vi "Secondary Xbox.vi"(10 "Secondary":T3, 11 "Dash Data In":T2={"Joy Stick"={"Primary"={"Buttons"={"A"=FALSE, "B"=FALSE, "X"=FALSE, "Y"=FALSE, "Left Bumper"=FALSE, "Right Bumper"=FALSE, "Back"=FALSE, "Start"=FALSE, "Left Thumbstick"=FALSE, "Right Thumbstick"=FALSE}, "Axes"={"Left Stick X "=0.0, "Left Stick Y"=0.0, "Triggers"=-0.0, "Right Stick X"=0.0, "Right Stick Y"=0.0, "D-Pad X"=0.0}}, "Secondary"={"Buttons"={"A"=FALSE, "B"=FALSE, "X"=FALSE, "Y"=FALSE, "Left Bumper"=FALSE, "Right Bumper"=FALSE, "Back"=FALSE, "Start"=FALSE, "Left Thumbstick"=FALSE, "Right Thumbstick"=FALSE}, "Axes"={"Left Stick X "=0.0, "Left Stick Y"=0.0, "Triggers"=0.0, "Right Stick X"=0.0, "Right Stick Y"=0.0, "D-Pad X"=0.0}}}, "Shooter"={"RPM Current"=0.0, "RPM Set"=0.0, "In Range?"=FALSE}, "Arm"={"Arm Current"=0.0, "Arm Set"=0.0, "At Position?"=FALSE, "Reset Encoder"=FALSE}, "Drive"={"Right"=0.0, "Left"=0.0}, "Climb State"=enum."Arm Attach", "Change Retical"=FALSE, "Solenoids"={"Robot Angle"=enum."Off", "Shooter Angle"=enum."Off", "Arm Lock"=enum."Off"}, "Shooter Speeds"=[]}) -> (3 "Dash Data Out 2":T2={"Joy Stick"={"Primary"={"Buttons"={"A"=FALSE, "B"=FALSE, "X"=FALSE, "Y"=FALSE, "Left Bumper"=FALSE, "Right Bumper"=FALSE, "Back"=FALSE, "Start"=FALSE, "Left Thumbstick"=FALSE, "Right Thumbstick"=FALSE}, "Axes"={"Left Stick X "=0.0, "Left Stick Y"=0.0, "Triggers"=-0.0, "Right Stick X"=0.0, "Right Stick Y"=0.0, "D-Pad X"=0.0}}, "Secondary"={"Buttons"={"A"=FALSE, "B"=FALSE, "X"=FALSE, "Y"=FALSE, "Left Bumper"=FALSE, "Right Bumper"=FALSE, "Back"=FALSE, "Start"=FALSE, "Left Thumbstick"=FALSE, "Right Thumbstick"=FALSE}, "Axes"={"Left Stick X "=0.0, "Left Stick Y"=0.0, "Triggers"=0.0, "Right Stick X"=0.0, "Right Stick Y"=0.0, "D-Pad X"=0.0}}}, "Shooter"={"RPM Current"=0.0, "RPM Set"=0.0, "In Range?"=FALSE}, "Arm"={"Arm Current"=0.0, "Arm Set"=0.0, "At Position?"=FALSE, "Reset Encoder"=FALSE}, "Drive"={"Right"=0.0, "Left"=0.0}, "Climb State"=enum."Arm Attach", "Change Retical"=FALSE, "Solenoids"={"Robot Angle"=enum."Off", "Shooter Angle"=enum."Off", "Arm Lock"=enum."Off"}, "Shooter Speeds"=[]})   [LabVIEW 2012]
uses:
  <vilib>/Rock Robotics/WPI/Solenoid/WPI_SolenoidValue.ctl
types:
  T1 = typedef "WPI_SolenoidValue.ctl" = enum16{"Off", "On", "Forward", "Reverse"}
  T2 = cluster{"Joy Stick":cluster{"Primary":cluster{"Buttons":cluster{"A":bool, "B":bool, "X":bool, "Y":bool, "Left Bumper":bool, "Right Bumper":bool, "Back":bool, "Start":bool, "Left Thumbstick":bool, "Right Thumbstick":bool}, "Axes":cluster{"Left Stick X ":dbl, "Left Stick Y":dbl, "Triggers":dbl, "Right Stick X":dbl, "Right Stick Y":dbl, "D-Pad X":dbl}}, "Secondary":cluster{"Buttons":cluster{"A":bool, "B":bool, "X":bool, "Y":bool, "Left Bumper":bool, "Right Bumper":bool, "Back":bool, "Start":bool, "Left Thumbstick":bool, "Right Thumbstick":bool}, "Axes":cluster{"Left Stick X ":dbl, "Left Stick Y":dbl, "Triggers":dbl, "Right Stick X":dbl, "Right Stick Y":dbl, "D-Pad X":dbl}}}, "Shooter":cluster{"RPM Current":dbl, "RPM Set":dbl, "In Range?":bool}, "Arm":cluster{"Arm Current":dbl, "Arm Set":dbl, "At Position?":bool, "Reset Encoder":bool}, "Drive":cluster{"Right":dbl, "Left":dbl}, "Climb State":enum16{"Arm Wait", "Arm Up", "Arm Down", "Arm Attach"}, "Change Retical":bool, "Solenoids":cluster{"Robot Angle":T1, "Shooter Angle":T1, "Arm Lock":T1}, "Shooter Speeds":dbl[]}
  T3 = cluster{"Buttons":cluster{"A":bool, "B":bool, "X":bool, "Y":bool, "Left Bumper":bool, "Right Bumper":bool, "Back":bool, "Start":bool, "Left Thumbstick":bool, "Right Thumbstick":bool}, "Axes":cluster{"Left Stick X ":dbl, "Left Stick Y":dbl, "Triggers":dbl, "Right Stick X":dbl, "Right Stick Y":dbl, "D-Pad X":dbl}}
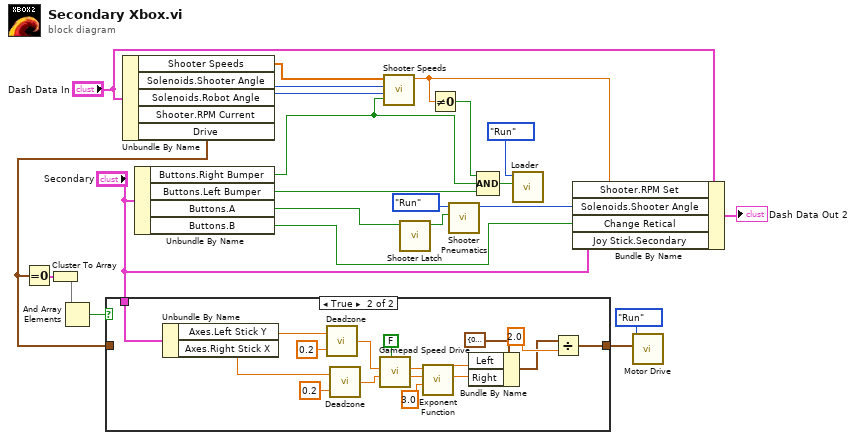
[diagram p0: block diagram]
diagram:
  n1 = Unbundle By Name("Dash Data In") -> ("Shooter Speeds"=w17:dbl[], "Solenoids.Shooter Angle"=w14:T1, "Solenoids.Robot Angle"=w16:T1, "Drive"=w8:cluster{"Right":dbl, "Left":dbl})  [unwired: 1 out]
  n2 = Equal To 0?(x=w8) -> (x = 0?=w9:cluster{"Right":bool, "Left":bool})
  n3 = Cluster To Array(cluster=w9) -> (array=w7:bool[])
  n4 = And Array Elements(Boolean array=w7) -> (logical AND=w6:bool)
  n5 = case shown="True" w6 {
    tunnel: "Secondary" -> [_ w30]
    tunnel: [w24 w26] -> w10
    tunnel: w8 -> [w24 _]
    frame False {
    }
    frame True {
      n6 = Unbundle By Name(w30) -> ("Axes.Left Stick Y"=w29:dbl, "Axes.Right Stick X"=w28:dbl)
      n7 = call "Deadzone.vi"("Deadzone"=0.2, "Input"=w29) -> ("Output"=w37:dbl)
      n8 = call "Deadzone.vi"("Deadzone"=0.2, "Input"=w28) -> ("Output"=w35:dbl)
      n9 = call "Gamepad Speed Drive.vi"("Quick Turn"=FALSE, "Turn"=w35, "Speed"=w37) -> ("Right Output"=w40:dbl, "Left Output"=w41:dbl)  [unwired: 7 in]
      n10 = call "Exponent Function.vi"("Exponent"=3.0, "Left In"=w40, "Right In"=w41) -> ("Right Out"=w32:dbl, "Left Out"=w33:dbl)  [unwired: 7 in]
      n11 = Bundle By Name(cluster=cluster{"Right":dbl, "Left":dbl} {"Right"=0.0, "Left"=0.0} ("Motor"), "Left"=w33, "Right"=w32) -> (w27:cluster{"Right":dbl, "Left":dbl})
      n12 = Divide(x=w27, y=2.0) -> (x/y=w26:cluster{"Right":dbl, "Left":dbl})
    }
  }
  n13 = Unbundle By Name("Secondary") -> ("Buttons.Right Bumper"=w5:bool, "Buttons.Left Bumper"=w3:bool, "Buttons.A"=w2:bool, "Buttons.B"=w1:bool)
  n14 = call "Shooter Speeds.vi"("Right Bumper"=w5, "Robot Angle"=w16, "Shooter Angle"=w14, "Shooter Speeds"=w17) -> ("f"=w15:dbl)  [unwired: 7 in]
  n15 = call "Shooter Latch.vi"("Input"=w2) -> ("Latched"=w23:bool)  [unwired: 10 in]
  n16 = Not Equal To 0?(x=w15) -> (x != 0?=w4:bool)
  n17 = call "Shooter Pneumatics.vi"("Boolean"=w23, "Enum"=enum16{"Start", "Run", "End"}."Run") -> ("Shooter Angle"=w20:T1)  [unwired: 9 in]
  n18 = Compound Arithmetic op=AND(w4, w5, w3) -> (w13:bool)
  n19 = call "Loader.vi"("Enum"=enum16{"Start", "Run", "End"}."Run", "Run"=w13) -> ()  [unwired: 9 in]
  n20 = Bundle By Name(cluster="Dash Data In", "Shooter.RPM Set"=w15, "Solenoids.Shooter Angle"=w20, "Change Retical"=w1, "Joy Stick.Secondary"="Secondary") -> (→"Dash Data Out 2":T2)
  n21 = call "Motor Drive.vi"("Motor"=w10, "Enum"=enum16{"Start", "Run", "End"}."Run") -> ()  [unwired: 10 in]
